vi "Clear Error (if UDP closed).vi"(10 "error in":errorcluster, 11 "udp refnum":refnum<k16>) -> (2 "error out":errorcluster, 5 "stop?":bool)   [LabVIEW 2017, in "Game.lvlib" / "GameComms.lvlib"]
uses:
  GameComms.lvlib
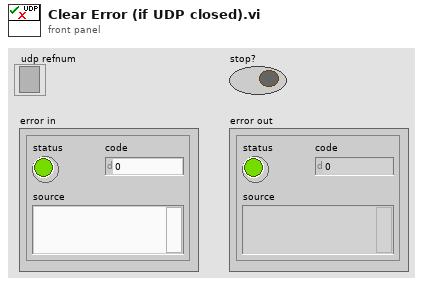
[diagram p1: front panel]
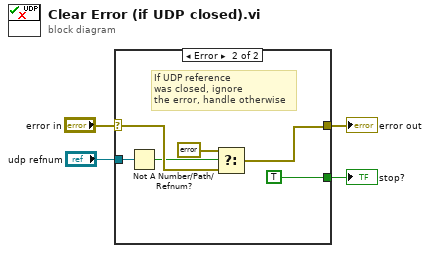
[diagram p0: block diagram]
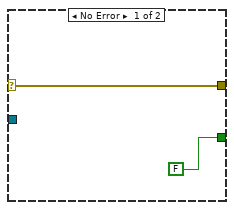
[diagram p2: hidden frame]
diagram:
  n1 = case shown="Error" "error in" {
    selector: "error in" -> [w6 w12]
    tunnel: "udp refnum" -> [_ w8]
    tunnel: [w6 w10] -> w3
    tunnel: [FALSE TRUE] -> w2
    frame No Error {
    }
    frame Error {
      # "If UDP reference\nwas closed, ignore\nthe error, handle otherwise"
      n2 = Not A Number/Path/Refnum?(number/path/refnum=w8) -> (NaN/Path/Refnum?=w7:bool)
      n3 = Select(t=errorcluster {"status"=FALSE, "code"=0, "source"=""}, s=w7, f=w12) -> (s? t:f=w10:errorcluster)
    }
  }
  "error out" <- w3
  "stop?" <- w2
